vi "LSX Clear Key Latch.vi"(8 "error in (no error)":errorcluster, 10 "lKey":i32, 11 "lLSID":i32) -> (0 "error out":errorcluster, 3 "function return":i32)   [LabVIEW 2018, in "Tango.lvlib"]
doc: "TANGOAPI int TANGOCALL LSX_ClearKeyLatch (int lLSID, int lKey);"
uses:
  Tango.lvlib
  SubVIs/Tango_DLL.dll
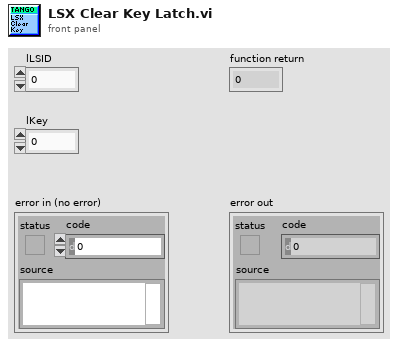
[diagram p1: front panel]
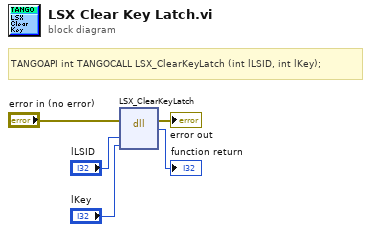
[diagram p0: block diagram]
diagram:
  # "TANGOAPI int TANGOCALL LSX_ClearKeyLatch (int lLSID, int lKey);"
  n1 = dll-call lib="C:/Users/Familie/Documents/LabviewIX81/lib/TANGO Stage/SubVIs/Tango_DLL.*" fn="LSX_ClearKeyLatch"(error in="error in (no error)", "lLSID"="lLSID", "lKey"="lKey") -> (error out=→"error out":errorcluster, →"function return":i32)  [unwired: 4 in, 1 out]
